vi "get freq byte.vi"(8 "error in (no error)":errorcluster caption="에러 입력(에러 없음)", 10 "freq":u32, 11 "DW7800 입력":refnum<class "DW7800.lvclass">) -> (0 "error out":errorcluster caption="에러 출력", 2 "byte value":u8 format="%02x", 3 "DW7800 출력":refnum<class "DW7800.lvclass">)   [LabVIEW 2020, in "DW7800.lvclass"]
uses:
  DW7800.lvclass
  1afa0ecb-7aff-4dfa-bf30-fac7acd1e500.vi
  <vilib>/Comparison/Equal/Equal Functor/Equal Functor.lvclass
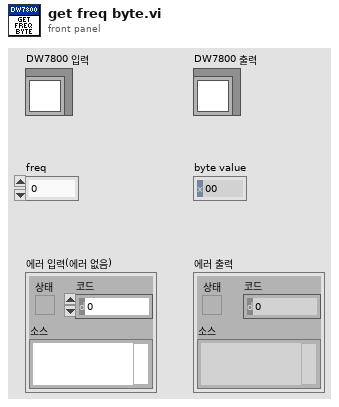
[diagram p1: front panel]
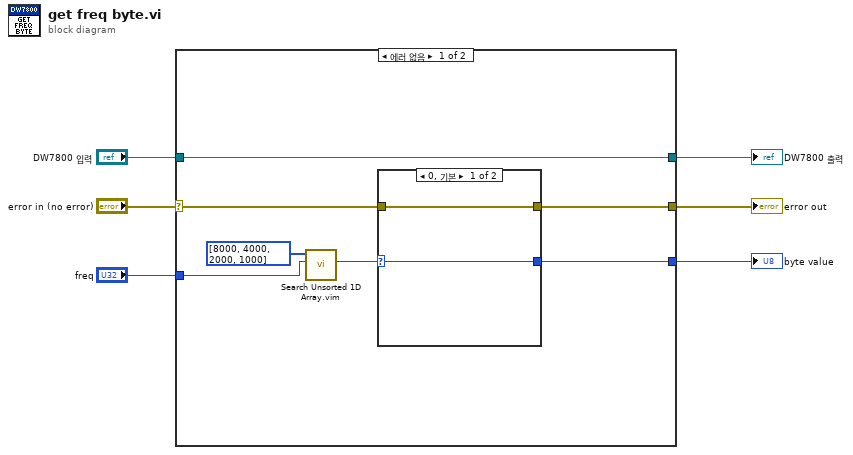
[diagram p0: block diagram]
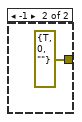
[diagram p2: hidden frame]
diagram:
  n1 = case shown="에러 없음" "error in (no error)" {
    selector: "error in (no error)" -> [w10 w18]
    tunnel: [w7 w18] -> w5
    tunnel: "DW7800 입력" -> [w13 w17]
    tunnel: [w13 w17] -> w3
    tunnel: "freq" -> [w11 _]
    tunnel: [w8 _] -> w1
    frame No Error {
      n2 = call "Search Unsorted 1D Array.vim"("element"=w11, "unsorted 1D array"=u32[] [8000, 4000, 2000, 1000]) -> ("index of element"=w9:i32)  [unwired: 9 in]
      n3 = case shown="0, 기본" w9 {
        selector: w9 -> [w15 _]
        tunnel: w10 -> [w14 _]
        tunnel: [w15 _] -> w8
        tunnel: [w14 errorcluster {"status"=TRUE, "code"=0, "source"=""} ("error IO")] -> w7
        frame 0, Default {
        }
        frame -1 {
        }
      }
    }
    frame Error {
    }
  }
  "error out" <- w5
  "DW7800 출력" <- w3
  "byte value" <- w1
